vi "Load Macro.vi"(7 "Macro Name":string, 8 "error in (no error)":errorcluster, 11 "refnum":T4) -> (0 "error out":errorcluster, 2 "Macro":T1, 3 "refnum out":T4)   [LabVIEW 2023]
uses:
  <vilib>/Utility/config.llb/Config Data RefNum.ctl
  CTLs/Macro Cluster v2.0.ctl
  CTLs/Step.ctl
  CTLs/Step Type.ctl
  CTLs/Macro Cluster v1.0.ctl
  <vilib>/Utility/config.llb/Read Key (String).vi
  <vilib>/Utility/config.llb/NI_LVConfig.lvlib
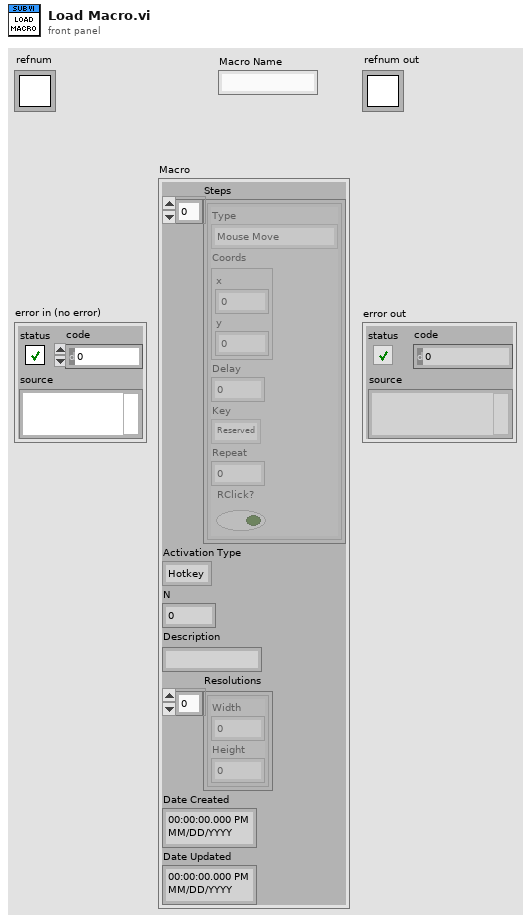
[diagram p1: front panel]
types:
  T1 = typedef "Macro Cluster v2.0.ctl" = cluster{"Steps":T2[], "Activation Type":enum32{"Hotkey", "Automatic"}, "N":i32, "Description":string, "Resolutions":cluster{"Width":i16, "Height":i16}[], "Date Created":timestamp, "Date Updated":timestamp}
  T2 = typedef "Step.ctl" = cluster{"Type":T3, "Coords":cluster{"x":i32, "y":i32}, "Delay":i32, "Key":u8, "Repeat":i32, "RClick?":bool}
  T3 = typedef "Step Type.ctl" = enum16{"Mouse Move", "Mouse Click", "Key Press", "Wait", "Mouse Down", "Mouse Up", "Key Down", "Key Up"}
  T4 = typedef "NI_LVConfig.lvlib/Config Data RefNum.ctl" = refnum<k1>
  T5 = typedef "Macro Cluster v1.0.ctl" = cluster{"Steps":T2[], "Activation Type":enum32{"Hotkey", "Automatic"}, "N":i32}
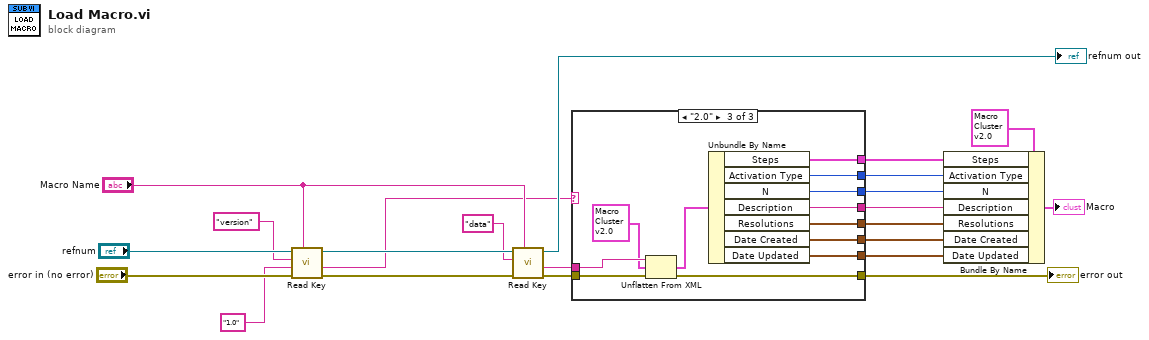
[diagram p0: block diagram]
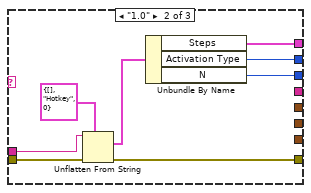
[diagram p3: hidden frame]
diagram:
  n1 = call-poly <vilib>:"Read Key.vi"("section"="Macro Name", "error in (no error)"="error in (no error)", "default value"="1.0", "key"="version", "refnum"="refnum") -> ("error out"=w14:errorcluster, "value"=w10:string, "refnum out"=w21:T4)  [unwired: 3 in, 1 out]
  n2 = call-poly <vilib>:"Read Key.vi"("section"="Macro Name", "error in (no error)"=w14, "key"="data", "refnum"=w21) -> ("error out"=w18:errorcluster, "value"=w19:string, "refnum out"=→"refnum out":T4)  [unwired: 4 in, 1 out]
  n3 = case shown="\"2.0\"" w10 {
    tunnel: w19 -> [_ w31 w43]
    tunnel: w18 -> [w23 w30 w42]
    tunnel: [w23 w29 w41] -> w2
    tunnel: [_ w27 w39] -> w9
    tunnel: [_ w26 w38] -> w8
    tunnel: [_ w25 w37] -> w7
    tunnel: [_ _ w35] -> w6
    tunnel: [_ _ w34] -> w5
    tunnel: [_ _ w33] -> w4
    tunnel: [_ _ w32] -> w3
    frame "False", Default {
    }
    frame "1.0" {
      n4 = Unflatten From String(type=T5 {"Steps"=[], "Activation Type"=enum."Hotkey", "N"=0} ("Macro Cluster"), binary string=w31, error in (no error)=w30) -> (value=w28:T5, error out=w29:errorcluster)  [unwired: 2 in, 1 out]
      n5 = Unbundle By Name(w28) -> ("Steps"=w27:T2[], "Activation Type"=w26:enum32{"Hotkey", "Automatic"}, "N"=w25:i32)
    }
    frame "2.0" {
      n6 = Unflatten From XML(xml string=w43, type=T1 {"Steps"=[], "Activation Type"=enum."Hotkey", "N"=0, "Description"="", "Resolutions"=[], "Date Created"=timestamp(0 s since 1904-01-01), "Date Updated"=timestamp(0 s since 1904-01-01)} ("Macro Cluster"), error in (no error)=w42) -> (value=w40:T1, error out=w41:errorcluster)
      n7 = Unbundle By Name(w40) -> ("Steps"=w39:T2[], "Activation Type"=w38:enum32{"Hotkey", "Automatic"}, "N"=w37:i32, "Description"=w35:string, "Resolutions"=w34:cluster{"Width":i16, "Height":i16}[], "Date Created"=w33:timestamp, "Date Updated"=w32:timestamp)
    }
  }
  "error out" <- w2
  n8 = Bundle By Name(cluster=T1 {"Steps"=[], "Activation Type"=enum."Hotkey", "N"=0, "Description"="", "Resolutions"=[], "Date Created"=timestamp(0 s since 1904-01-01), "Date Updated"=timestamp(0 s since 1904-01-01)} ("Macro Cluster"), "Steps"=w9, "Activation Type"=w8, "N"=w7, "Description"=w6, "Resolutions"=w5, "Date Created"=w4, "Date Updated"=w3) -> (→"Macro":T1)
